vi "tcpip_forward.vi"() -> ()   [LabVIEW 2013]
uses:
  <vilib>/Utility/error.llb/DialogType.ctl
  libssh2/libssh2_init_default.vi
  libssh2/libssh2_session_handshake_tcp.vi
  libssh2/libssh2.lvlib
panel:
  in  "stop":bool
  in  "local_destport":i32=4444
  in  "local_destip":string="localhost"
  in  "remote_wantport":i32=2222
  in  "remote_listenhost":string="localhost"
  in  "server_ip":string="127.0.0.1"
  in  "password":string
  in  "username":string
  out "error out":errorcluster
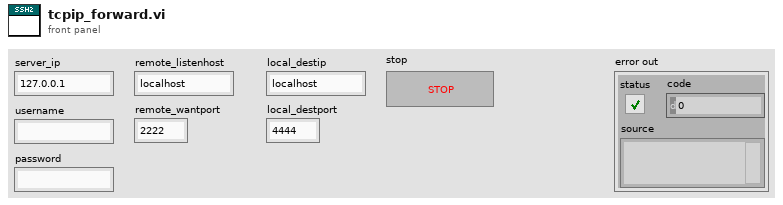
[diagram p1: front panel]
types:
  T1 = typedef "libssh2.lvlib/Session Refnum.ctl" = refnum<k1>
  T2 = typedef "libssh2.lvlib/Listener Refnum.ctl" = refnum<k1>
  T3 = typedef "libssh2.lvlib/Channel Refnum.ctl" = refnum<k1>
  T4 = enum16{"Standard", "Buffered", "CRLF", "Immediate"}
  T5 = typedef "DialogType.ctl" = u16
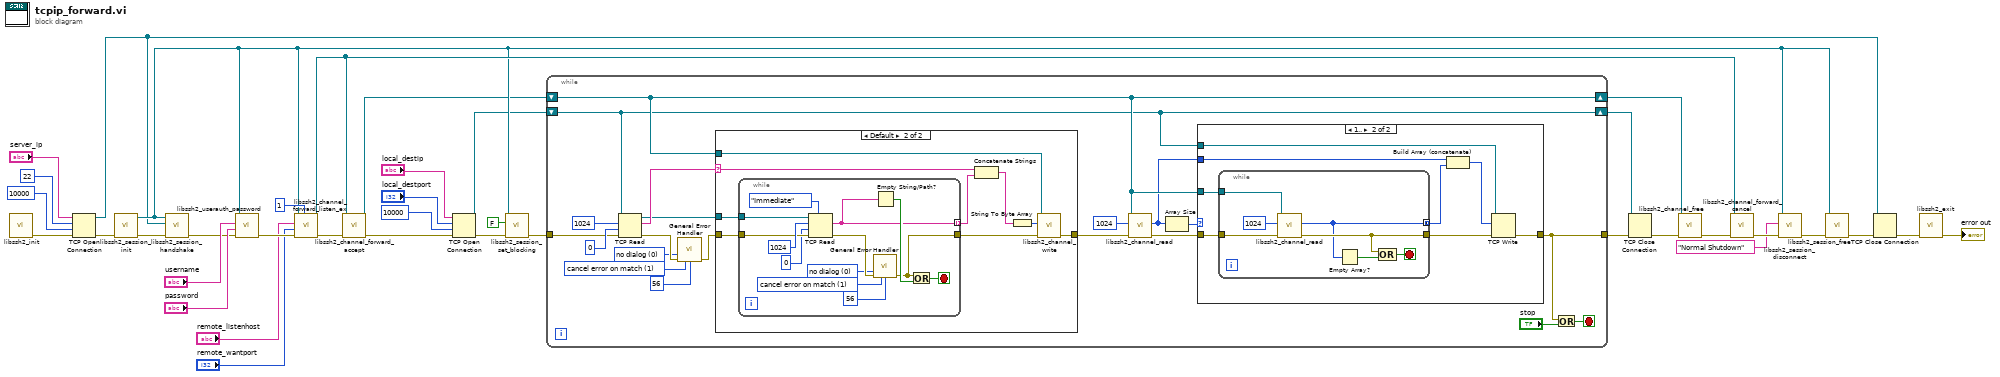
[diagram p0: block diagram]
diagram:
  n1 = call-poly "libssh2_init.vi"() -> ("error out"=w34:errorcluster)  [unwired: 11 in]
  n2 = TCP Open Connection(address="server_ip", remote port or service name=u16 22, timeout ms (60000)=10000, error in (no error)=w34) -> (connection ID=w1:refnum<k5>, error out=w2:errorcluster)  [unwired: 1 in]
  n3 = call "libssh2_session_init.vi"("error in (no error)"=w2) -> ("error out"=w33:errorcluster, "session"=w9:T1)  [unwired: 9 in]
  n4 = call-poly "libssh2_session_handshake.vi"("error in (no error)"=w33, "tcp connection"=w1, "session"=w9) -> ("error out"=w12:errorcluster)  [unwired: 8 in]
  n5 = call "libssh2_userauth_password.vi"("error in (no error)"=w12, "password"="password", "username"="username", "session"=w9) -> ("error out"=w31:errorcluster)  [unwired: 7 in]
  n6 = call "libssh2_channel_forward_listen_ex.vi"("queue_maxsize"=1, "error in (no error)"=w31, "port"="remote_wantport", "host"="remote_listenhost", "session"=w9) -> ("error out"=w27:errorcluster, "listener"=w22:T2)  [unwired: 4 in, 1 out]
  n7 = call "libssh2_channel_forward_accept.vi"("error in (no error)"=w27, "listener"=w22) -> ("error out"=w26:errorcluster, "channel"=w6:T3)  [unwired: 8 in]
  n8 = TCP Open Connection(address="local_destip", remote port or service name="local_destport", timeout ms (60000)=10000, error in (no error)=w26) -> (connection ID=w5:refnum<k5>, error out=w11:errorcluster)  [unwired: 1 in]
  n9 = call "libssh2_session_set_blocking.vi"("error in (no error)"=w11, "blocking"=FALSE, "session"=w9) -> ("error out"=w10:errorcluster)  [unwired: 8 in]
  n10 = while {
    tunnel: w10 -> [w48]
    tunnel: [w44] -> w4
    shift-right: [w50] -> w8
    shift-left: w6 -> [w50]
    shift-right: [w45] -> w7
    shift-left: w5 -> [w45]
    stop <- w42 stop-if-true
    w39 = T5 0 items=["no dialog", "OK message", "continue or stop message", "OK message + warnings", "continue/stop + warnings"] ("type of dialog (OK msg:1)")
    w41 = 1 items=["no exception", "cancel error on match", "set error on match"] ("[exception action] (none:0)")
    n11 = TCP Read(connection ID=w45, bytes to read=1024, error in (no error)=w48, 9:0 ("timeout ms (25000)")) -> (connection ID out=w46:refnum<k5>, data out=w56:string, error out=w49:errorcluster)  [unwired: 1 in]
    n12 = call <vilib>:"General Error Handler.vi"("type of dialog (OK msg:1)"=w39, "error in (no error)"=w49, "[exception action] (none:0)"=w41, "[exception code]"=56 ("specific error code to clear (0: all)")) -> ("error out"=w47:errorcluster)  [unwired: 7 in, 4 out]
    n13 = case shown="Default" w56 {
      selector: w56 -> [_ w77]
      tunnel: [w74 w80] -> w52
      tunnel: w46 -> [_ w83]
      tunnel: w47 -> [w74 w82]
      tunnel: w50 -> [_ w79]
      frame "" {
      }
      frame Default {
        n14 = while {
          tunnel: [w88] -> w81
          tunnel: w83 -> [w94]
          tunnel: w82 -> [w91]
          tunnel: [w87] -> w78 mode=indexing
          stop <- w92 stop-if-true
          w84 = T5 0 items=["no dialog", "OK message", "continue or stop message", "OK message + warnings", "continue/stop + warnings"] ("type of dialog (OK msg:1)")
          w85 = 1 items=["no exception", "cancel error on match", "set error on match"] ("[exception action] (none:0)")
          n15 = TCP Read(connection ID=w94, bytes to read=1024, error in (no error)=w91, 7:T4."Immediate" ("mode (standard)"), 9:0 ("timeout ms (25000)")) -> (data out=w87:string, error out=w89:errorcluster)  [unwired: 1 out]
          n16 = call <vilib>:"General Error Handler.vi"("type of dialog (OK msg:1)"=w84, "error in (no error)"=w89, "[exception action] (none:0)"=w85, "[exception code]"=56 ("specific error code to clear (0: all)")) -> ("error out"=w88:errorcluster)  [unwired: 7 in, 4 out]
          n17 = Empty String/Path?(string/path=w87) -> (empty?=w93:bool)
          n18 = Or(x=w88, y=w93) -> (x .or. y?=w92:bool)
        }
        n19 = Concatenate Strings(w77, w78) -> (w76:string)
        n20 = String To Byte Array(string=w76) -> (unsigned byte array=w75:u8[])
        n21 = call "libssh2_channel_write.vi"("error in (no error)"=w81, "buffer"=w75, "channel"=w79) -> ("error out"=w80:errorcluster)  [unwired: 7 in, 1 out]
      }
    }
    n22 = call "libssh2_channel_read.vi"("error in (no error)"=w52, "buffer length"=1024 ("buflen"), "channel"=w50) -> ("error out"=w51:errorcluster, "buffer"=w38:u8[])  [unwired: 7 in]
    n23 = Array Size(array=w38) -> (size(s)=w54:i32)
    n24 = case shown="1.." w54 {
      tunnel: [w58 w64] -> w44
      tunnel: w50 -> [_ w66]
      tunnel: w45 -> [_ w63]
      tunnel: w51 -> [w58 w65]
      tunnel: w38 -> [_ w62]
      frame Default {
      }
      frame 1.. {
        n25 = while {
          tunnel: w66 -> [w69]
          tunnel: w65 -> [w70]
          tunnel: [w67] -> w61 mode=concatenating
          tunnel: [w68] -> w59
          stop <- w73 stop-if-true
          n26 = call "libssh2_channel_read.vi"("error in (no error)"=w70, "buffer length"=1024 ("buflen"), "channel"=w69) -> ("error out"=w68:errorcluster, "buffer"=w67:u8[])  [unwired: 7 in]
          n27 = Empty Array?(array=w67) -> (empty?=w72:bool)
          n28 = Compound Arithmetic op=OR(w68, w72) -> (w73:bool)
        }
        n29 = Build Array (concatenate)(w62, w61) -> (w60:u8[])
        n30 = TCP Write(connection ID=w63, data in=w60, error in (no error)=w59) -> (error out=w64:errorcluster)  [unwired: 1 in, 2 out]
      }
    }
    n31 = Or(x=w44, y="stop") -> (x .or. y?=w42:bool)
  }
  n32 = TCP Close Connection(connection ID=w7, error in (no error)=w4) -> (error out=w20:errorcluster)  [unwired: 1 in, 1 out]
  n33 = call "libssh2_channel_free.vi"("error in (no error)"=w20, "channel"=w8) -> ("error out"=w23:errorcluster)  [unwired: 9 in]
  n34 = call "libssh2_channel_forward_cancel.vi"("error in (no error)"=w23, "listener"=w22) -> ("error out"=w21:errorcluster)  [unwired: 9 in]
  n35 = call "libssh2_session_disconnect.vi"("error in (no error)"=w21, "description"="Normal Shutdown", "session"=w9) -> ("error out"=w32:errorcluster)  [unwired: 8 in]
  n36 = call "libssh2_session_free.vi"("error in (no error)"=w32, "session"=w9) -> ("error out"=w13:errorcluster)  [unwired: 9 in]
  n37 = TCP Close Connection(connection ID=w1, error in (no error)=w13) -> (error out=w15:errorcluster)  [unwired: 1 in, 1 out]
  n38 = call "libssh2_exit.vi"("error in (no error)"=w15) -> ("error out"=→"error out":errorcluster)  [unwired: 10 in]
